vi "STSatZ_createHeader (SubVI).vi"(4 "Current":sgl, 5 "TipOffset":sgl, 6 "Bias":sgl, 7 "z range":dbl, 8 "error in (no error)":errorcluster, 9 "points":i32, 10 "z step":dbl, 11 "Application in":refnum<vi>) -> (0 "error out":errorcluster, 2 "File ref":refnum<file>, 3 "Application out":refnum<vi>)   [LabVIEW 2014]
uses:
  <userlib>/Nanonis Prog Interface V5/Nanonis Prog Interface.lvlib
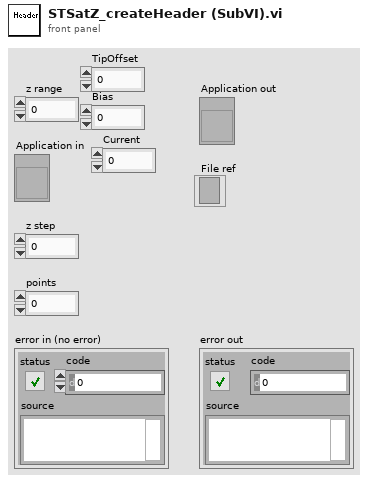
[diagram p1: front panel]
types:
  T1 = cluster{"center X (m)":sgl, "center Y (m)":sgl, "width (m)":sgl, "height (m)":sgl, "angle (deg)":sgl}
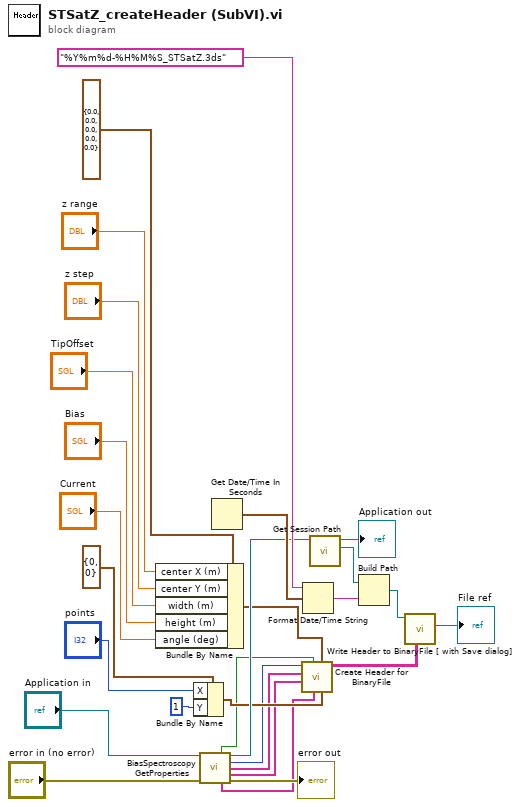
[diagram p0: block diagram]
diagram:
  n1 = Bundle By Name(cluster=T1 {"center X (m)"=0.0, "center Y (m)"=0.0, "width (m)"=0.0, "height (m)"=0.0, "angle (deg)"=0.0} ("Grid param"), "center X (m)"="z range", "center Y (m)"="z step", "width (m)"="TipOffset", "height (m)"="Bias", "angle (deg)"="Current") -> (w15:T1)
  n2 = Bundle By Name(cluster=cluster{"X":i32, "Y":i32} {"X"=0, "Y"=0} ("Grid points"), "X"="points", "Y"=1) -> (w12:cluster{"X":i32, "Y":i32})
  n3 = call <userlib>:"BiasSpectroscopy GetProperties.vi"("Application ref in"="Application in", "Error in (no error)"="error in (no error)") -> ("Backward sweep"=w8:bool, "Application ref out"=w20:refnum<vi>, "Number of points"=w7:i32, "Channels"=w5:string[], "Parameters"=w4:string[], "Fixed parameters"=w6:string[], "Error out"=→"error out":errorcluster)  [unwired: 5 in, 2 out]
  n4 = Get Date/Time In Seconds() -> (seconds since 1Jan1904=w24:timestamp)
  n5 = call <userlib>:"Create Header for BinaryFile.vi"("Grid points"=w12, "Grid param"=w15, "Fixed parameters"=w6, "Backward sweep"=w8, "Parameters"=w4, "Channels"=w5, "Points per sweep"=w7) -> ("Header (fixed attributes)"=w9:string[][])  [unwired: 4 in]
  n6 = Format Date/Time String(time format string (%c)="%Y%m%d-%H%M%S_STSatZ.3ds", seconds (now)=w24) -> (date/time string=w26:string)  [unwired: 1 in]
  n7 = call <userlib>:"Get Session Path.vi"("Application ref in"=w20) -> ("Session path"=w22:path, "Application ref out"=→"Application out":refnum<vi>)  [unwired: 8 in, 1 out]
  n8 = Build Path(base path=w22, name or relative path=w26) -> (appended path=w23:path)
  n9 = call <userlib>:"Write Header to BinaryFile [ with Save dialog].vi"("Fixed Attributes"=w9, "Filename"=w23) -> ("File ref"=→"File ref":refnum<file>)  [unwired: 6 in, 3 out]
